vi "InitFromXML.vi"(8 "error in (no error)":errorcluster, 10 "XML":string, 11 "ClickableText in":refnum<class "ClickableText.lvclass">) -> (0 "error out":errorcluster, 3 "ClickableText out":refnum<class "ClickableText.lvclass">)   [LabVIEW 2009, in "NavScreen.lvlib" / "ClickableText.lvclass"]
uses:
  ClickableText.lvclass
  Link/Link.lvclass
  ItemData_Type.ctl
  ClickableText.lvclass/ClickableText.ctl
  NavScreen.lvlib
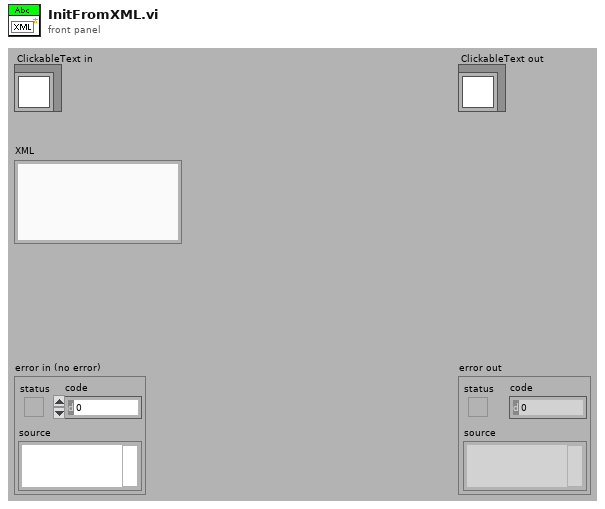
[diagram p1: front panel]
types:
  T1 = typedef "NavScreen.lvlib/ItemData_Type.ctl" = enum16{"None", "Folder", "New Project", "New VI", "Find", "VI", "Project", "New from template", "RT Project Wizard", "PDA Project Wizard", "Control", "Library", "Class", "XControl", "Runtime menu"}
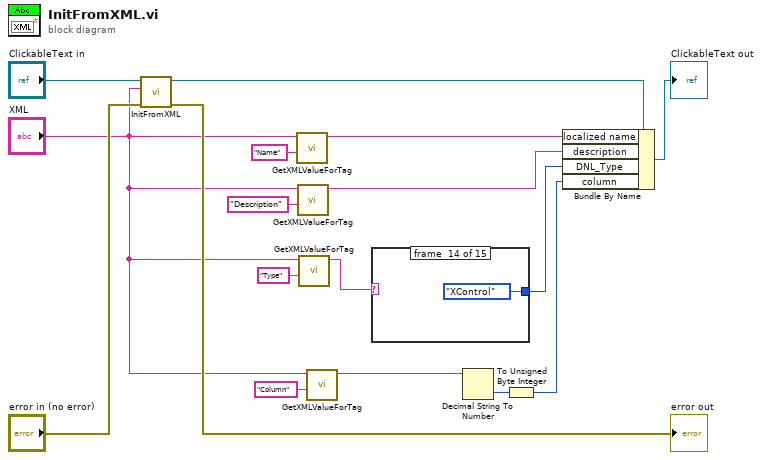
[diagram p0: block diagram]
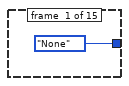
[diagram p2: hidden frame]
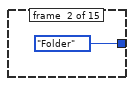
[diagram p3: hidden frame]
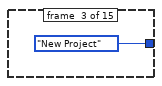
[diagram p4: hidden frame]
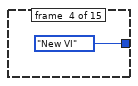
[diagram p5: hidden frame]
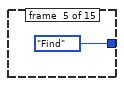
[diagram p6: hidden frame]
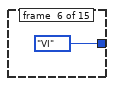
[diagram p7: hidden frame]
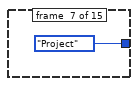
[diagram p8: hidden frame]
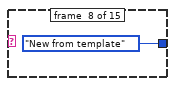
[diagram p9: hidden frame]
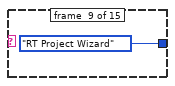
[diagram p10: hidden frame]
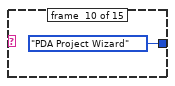
[diagram p11: hidden frame]
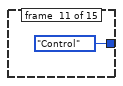
[diagram p12: hidden frame]
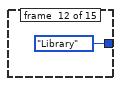
[diagram p13: hidden frame]
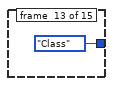
[diagram p14: hidden frame]
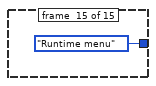
[diagram p15: hidden frame]
diagram:
  n1 = call-parent "InitFromXML.vi"("error in (no error)"="error in (no error)", "XML"="XML", "Link in"="ClickableText in") -> ("error out"=→"error out":errorcluster, "Link out"=w1:refnum<class "ClickableText.lvclass">)  [unwired: 7 in]
  n2 = call "GetXMLValueForTag.vi"("tag"="Name", "XML"="XML") -> ("value"=w14:string)  [unwired: 8 in, 1 out]
  n3 = call "GetXMLValueForTag.vi"("tag"="Description", "XML"="XML") -> ("value"=w12:string)  [unwired: 8 in, 1 out]
  n4 = call "GetXMLValueForTag.vi"("tag"="Type", "XML"="XML") -> ("value"=w9:string)  [unwired: 8 in, 1 out]
  n5 = call "GetXMLValueForTag.vi"("tag"="Column", "XML"="XML") -> ("value"=w6:string)  [unwired: 8 in, 1 out]
  n6 = case shown="\"PDA Project Wizard\"" w9 {
    tunnel: [ItemData_Type."None" ("DNL_Type") ItemData_Type."Folder" ("DNL_Type") ItemData_Type."New Project" ("DNL_Type") ItemData_Type."New VI" ("DNL_Type") ItemData_Type."Find" ("DNL_Type") ItemData_Type."VI" ("DNL_Type") ItemData_Type."Project" ("DNL_Type") ItemData_Type."New from template" ("DNL_Type") ItemData_Type."RT Project Wizard" ("DNL_Type") ItemData_Type."PDA Project Wizard" ("DNL_Type") ItemData_Type."Control" ("DNL_Type") ItemData_Type."Library" ("DNL_Type") ItemData_Type."Class" ("DNL_Type") ItemData_Type."XControl" ("DNL_Type") ItemData_Type."Runtime menu" ("DNL_Type")] -> w8
    frame #0 {
    }
    frame #1 {
    }
    frame #2 {
    }
    frame #3 {
    }
    frame #4 {
    }
    frame #5 {
    }
    frame #6 {
    }
    frame #7 {
    }
    frame #8 {
    }
    frame #9 {
    }
    frame #10 {
    }
    frame #11 {
    }
    frame #12 {
    }
    frame #13 {
    }
    frame #14 {
    }
  }
  n7 = Decimal String To Number(string=w6) -> (number=w5:i32)  [unwired: 2 in, 1 out]
  n8 = To Unsigned Byte Integer(number=w5) -> (unsigned 8bit integer=w3:u8)
  n9 = Bundle By Name(cluster=w1, "localized name"=w14, "description"=w12, "DNL_Type"=w8, "column"=w3) -> (→"ClickableText out":refnum<class "ClickableText.lvclass">)
